vi "Actor Core.vi"(8 "error in":errorcluster, 11 "Task_Abstr in":refnum<class "Task_Abstr.lvclass">) -> (0 "error out":errorcluster, 3 "Actor out":refnum<class "Actor.lvclass">)   [LabVIEW 2025, in "Task_Abstr.lvlib" / "Task_Abstr.lvclass"]
doc: "<p>(<strong>Filename</strong>: <span class=\"dnl\">Actor Framework.lvlib:Actor.lvclass:Actor Core.vi</span>)</p>\n<p>Receives messages to the actor, reacts to them, and initiates any error handling that may shut the actor down.</p>\n<p>Descendant classes may override this VI to append parallel tasks for the actor to complete while it handles messages. Overrides use the <a href=\"nihelplauncher://docs/csh?context=lvcore_glang_udclass\">Call Parent Class Method</a> node.</p>"
uses:
  Task_Abstr.lvclass
  C:/Program Files (x86)/National Instruments/LabVIEW 2025/vi.lib/ActorFramework/Actor/Actor.lvclass
  <vilib>/ActorFramework/Actor/Actor.lvclass
  Task_Abstr Messages/ReadData Msg/ReadData Msg.lvclass
  C:/Program Files (x86)/National Instruments/LabVIEW 2025/vi.lib/ActorFramework/Message/Message.lvclass
  <vilib>/ActorFramework/Actor/Actor.lvclass/Actor.ctl
  <vilib>/ActorFramework/Message Enqueuer/Message Enqueuer.lvclass/Message Enqueuer.ctl
  Task_Abstr.lvclass/Task_Abstr.ctl
  <vilib>/ActorFramework/Message Enqueuer/Init from Existing Queue.vi
  <vilib>/ActorFramework/Message Enqueuer/Message Enqueuer.lvclass
  <vilib>/ActorFramework/Actor Framework.lvlib
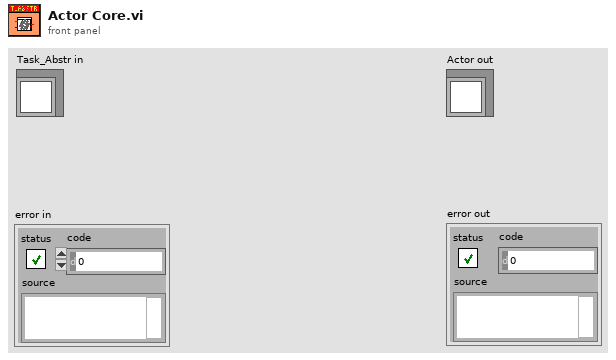
[diagram p1: front panel]
types:
  T1 = typedef "DAQ_Module.lvlib/DAQ_Module.lvclass/DAQ_Task_Config.ctl" = cluster{"TaskType":T2, "PhysicalChannels":string, "SampleRateConfiguration":cluster{"SampleRate":dbl, "SamplesPerChannel":u32, "SamplesPerRead":i32, "SampleMode":i32, "Clock Source":string}, "ChannelConfig":string}
  T2 = typedef "DAQ_Module.lvlib/DAQ_Module.lvclass/DAQ_Task_Type.ctl" = enum16{"AI", "Linear", "Angular", "AO"}
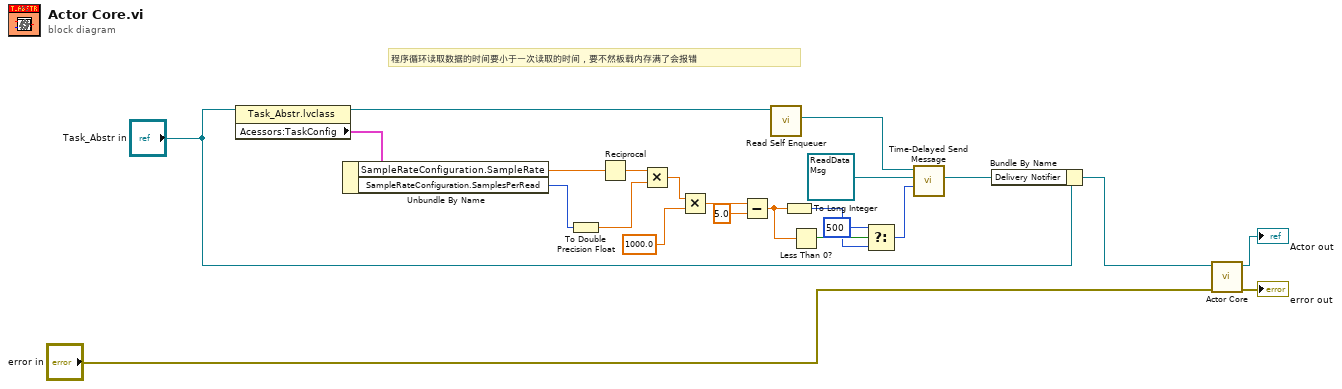
[diagram p0: block diagram]
diagram:
  # "程序循环读取数据的时间要小于一次读取的时间，要不然板载内存满了会报错"
  n1 = property class="Task_Abstr.lvclass"(reference="Task_Abstr in") -> (reference out=w18:refnum<class "Task_Abstr.lvclass">, "Acessors:TaskConfig"=w17:T1)  [unwired: 1 in, 1 out]
  n2 = Unbundle By Name(w17) -> ("SampleRateConfiguration.SampleRate"=w15:dbl, "SampleRateConfiguration.SamplesPerRead"=w16:i32)
  n3 = To Double Precision Float(number=w16) -> (double precision float=w13:dbl)
  n4 = Reciprocal(x=w15) -> (1/x=w14:dbl)
  n5 = Multiply(x=w14, y=w13) -> (x*y=w12:dbl)
  n6 = Multiply(x=w12, y=1000.0) -> (x*y=w10:dbl)
  n7 = Subtract(x=w10, y=5.0) -> (x-y=w5:dbl)
  n8 = call <vilib>:"Read Self Enqueuer.vi"("Actor"=w18) -> ("Self Enqueuer"=w19:refnum<class "Message Enqueuer.lvclass">)  [unwired: 10 in]
  n9 = To Long Integer(number=w5) -> (32bit integer=w3:i32)
  n10 = Less Than 0?(x=w5) -> (x < 0?=w4:bool)
  n11 = Select(t=500, s=w4, f=w3) -> (s? t:f=w1:i32)
  n12 = call <vilib>:"Time-Delayed Send Message.vi"("Milliseconds To Wait"=w1, "Message"=refnum<class "ReadData Msg.lvclass"> refnum ("Task_Abstr.lvlib:ReadData Msg.lvclass"), "Message Enqueuer"=w19) -> ("Delivery Notifier"=w7:refnum<notifier>)  [unwired: 7 in, 1 out]
  n13 = Bundle By Name(cluster="Task_Abstr in", "Delivery Notifier"=w7) -> (w6:refnum<class "Task_Abstr.lvclass">)
  n14 = call-parent "Actor Core.vi"("error in"="error in", "Actor in"=w6) -> ("error out"=→"error out":errorcluster, "Actor out"=→"Actor out":refnum<class "Actor.lvclass">)  [unwired: 8 in]
